vi "Mod_OFDM_Examine_OFDM_Symbol.vi"(0 "Configuration in":variant=variant("Data Source Pool "=variant(cluster{"mode (PN)":enum16{"PN", "pattern", "user"}, "PN sequence order (9)":i32, "base bit pattern (00001111)":enum16{"0", "1", "01", "0011", "00001111"}, "User base bit pattern":i8[]}[] [{"mode (PN)"=enum."PN", "PN sequence order (9)"=9, "base bit pattern (00001111)"=enum."00001111", "User base bit pattern"=[]}, {"mode (PN)"=enum."PN", "PN sequence order (9)"=9, "base bit pattern (00001111)"=enum."00001111", "User base bit pattern"=[]}, {"mode (PN)"=enum."PN", "PN sequence order (9)"=9, "base bit pattern (00001111)"=enum."00001111", "User base bit pattern"=[]}, {"mode (PN)"=enum."PN", "PN sequence order (9)"=9, "base bit pattern (00001111)"=enum."00001111", "User base bit pattern"=[]}, {"mode (PN)"=enum."PN", "PN sequence order (9)"=9, "base bit pattern (00001111)"=enum."00001111", "User base bit pattern"=[]}, {"mode (PN)"=enum."PN", "PN sequence order (9)"=9, "base bit pattern (00001111)"=enum."00001111", "User base bit pattern"=[]}]), "Modulator Source Pool "=variant(cluster{"M-QAM":enum16{"4", "16", "64", "256", "1024"}, "M-PSK":enum16{"2", "4", "8", "16", "32", "64", "128", "256"}, "Type of Modulation":enum16{"PSK", "QAM"}, "PSK":cluster{"differential PSK":enum16{"disable", "enable"}, "PSK type":u16}}[] [{"M-QAM"=enum."4", "M-PSK"=enum."4", "Type of Modulation"=enum."PSK", "PSK"={"differential PSK"=enum."disable", "PSK type"=0}}, {"M-QAM"=enum."4", "M-PSK"=enum."4", "Type of Modulation"=enum."PSK", "PSK"={"differential PSK"=enum."disable", "PSK type"=0}}, {"M-QAM"=enum."4", "M-PSK"=enum."4", "Type of Modulation"=enum."PSK", "PSK"={"differential PSK"=enum."disable", "PSK type"=0}}, {"M-QAM"=enum."4", "M-PSK"=enum."4", "Type of Modulation"=enum."PSK", "PSK"={"differential PSK"=enum."disable", "PSK type"=0}}, {"M-QAM"=enum."4", "M-PSK"=enum."4", "Type of Modulation"=enum."PSK", "PSK"={"differential PSK"=enum."disable", "PSK type"=0}}, {"M-QAM"=enum."4", "M-PSK"=enum."2", "Type of Modulation"=enum."PSK", "PSK"={"differential PSK"=enum."disable", "PSK type"=0}}]), "OFDM SYMBOL POOL"=variant(string[] []), "Sub Carrier Selection"=variant(cluster{"Sub Carrier":bool, "Data Source":u16, "Modulator":u16}[] [{"Sub Carrier"=TRUE, "Data Source"=0, "Modulator"=0}, {"Sub Carrier"=TRUE, "Data Source"=0, "Modulator"=0}, {"Sub Carrier"=TRUE, "Data Source"=0, "Modulator"=0}, {"Sub Carrier"=TRUE, "Data Source"=0, "Modulator"=0}, {"Sub Carrier"=TRUE, "Data Source"=0, "Modulator"=0}, {"Sub Carrier"=TRUE, "Data Source"=0, "Modulator"=0}, {"Sub Carrier"=TRUE, "Data Source"=0, "Modulator"=0}, {"Sub Carrier"=TRUE, "Data Source"=0, "Modulator"=0}, {"Sub Carrier"=TRUE, "Data Source"=0, "Modulator"=0}, {"Sub Carrier"=TRUE, "Data Source"=0, "Modulator"=0}, {"Sub Carrier"=TRUE, "Data Source"=0, "Modulator"=0}, {"Sub Carrier"=TRUE, "Data Source"=0, "Modulator"=0}, {"Sub Carrier"=TRUE, "Data Source"=0, "Modulator"=0}, {"Sub Carrier"=TRUE, "Data Source"=0, "Modulator"=0}, {"Sub Carrier"=TRUE, "Data Source"=0, "Modulator"=0}, {"Sub Carrier"=TRUE, "Data Source"=0, "Modulator"=0}, {"Sub Carrier"=TRUE, "Data Source"=0, "Modulator"=0}, {"Sub Carrier"=TRUE, "Data Source"=0, "Modulator"=0}, {"Sub Carrier"=TRUE, "Data Source"=0, "Modulator"=0}, {"Sub Carrier"=TRUE, "Data Source"=0, "Modulator"=0}, {"Sub Carrier"=TRUE, "Data Source"=0, "Modulator"=0}, {"Sub Carrier"=TRUE, "Data Source"=0, "Modulator"=0}, {"Sub Carrier"=TRUE, "Data Source"=0, "Modulator"=0}, {"Sub Carrier"=TRUE, "Data Source"=0, "Modulator"=0}, {"Sub Carrier"=TRUE, "Data Source"=0, "Modulator"=0}, {"Sub Carrier"=TRUE, "Data Source"=0, "Modulator"=0}, {"Sub Carrier"=TRUE, "Data Source"=0, "Modulator"=0}, {"Sub Carrier"=TRUE, "Data Source"=0, "Modulator"=0}, {"Sub Carrier"=TRUE, "Data Source"=0, "Modulator"=0}, {"Sub Carrier"=TRUE, "Data Source"=0, "Modulator"=0}, {"Sub Carrier"=TRUE, "Data Source"=0, "Modulator"=0}, {"Sub Carrier"=TRUE, "Data Source"=0, "Modulator"=0}, {"Sub Carrier"=TRUE, "Data Source"=0, "Modulator"=0}, {"Sub Carrier"=TRUE, "Data Source"=0, "Modulator"=0}, {"Sub Carrier"=TRUE, "Data Source"=0, "Modulator"=0}, {"Sub Carrier"=TRUE, "Data Source"=0, "Modulator"=0}, {"Sub Carrier"=TRUE, "Data Source"=0, "Modulator"=0}, {"Sub Carrier"=TRUE, "Data Source"=0, "Modulator"=0}, {"Sub Carrier"=TRUE, "Data Source"=0, "Modulator"=0}, {"Sub Carrier"=TRUE, "Data Source"=0, "Modulator"=0}, {"Sub Carrier"=TRUE, "Data Source"=0, "Modulator"=0}, {"Sub Carrier"=TRUE, "Data Source"=0, "Modulator"=0}, {"Sub Carrier"=TRUE, "Data Source"=0, "Modulator"=0}, {"Sub Carrier"=TRUE, "Data Source"=0, "Modulator"=0}, {"Sub Carrier"=TRUE, "Data Source"=0, "Modulator"=0}, {"Sub Carrier"=TRUE, "Data Source"=0, "Modulator"=0}, {"Sub Carrier"=TRUE, "Data Source"=0, "Modulator"=0}, {"Sub Carrier"=TRUE, "Data Source"=0, "Modulator"=0}, {"Sub Carrier"=TRUE, "Data Source"=0, "Modulator"=0}, {"Sub Carrier"=TRUE, "Data Source"=0, "Modulator"=0}, {"Sub Carrier"=TRUE, "Data Source"=0, "Modulator"=0}, {"Sub Carrier"=TRUE, "Data Source"=0, "Modulator"=0}, {"Sub Carrier"=TRUE, "Data Source"=0, "Modulator"=0}, {"Sub Carrier"=TRUE, "Data Source"=0, "Modulator"=0}, {"Sub Carrier"=TRUE, "Data Source"=0, "Modulator"=0}, {"Sub Carrier"=TRUE, "Data Source"=0, "Modulator"=0}, {"Sub Carrier"=TRUE, "Data Source"=0, "Modulator"=0}, {"Sub Carrier"=TRUE, "Data Source"=0, "Modulator"=0}, {"Sub Carrier"=TRUE, "Data Source"=0, "Modulator"=0}, {"Sub Carrier"=TRUE, "Data Source"=0, "Modulator"=0}, {"Sub Carrier"=TRUE, "Data Source"=0, "Modulator"=0}, {"Sub Carrier"=TRUE, "Data Source"=0, "Modulator"=0}, {"Sub Carrier"=TRUE, "Data Source"=0, "Modulator"=0}, {"Sub Carrier"=TRUE, "Data Source"=0, "Modulator"=0}, {"Sub Carrier"=TRUE, "Data Source"=0, "Modulator"=0}, {"Sub Carrier"=TRUE, "Data Source"=0, "Modulator"=0}, {"Sub Carrier"=TRUE, "Data Source"=0, "Modulator"=0}, {"Sub Carrier"=TRUE, "Data Source"=0, "Modulator"=0}, {"Sub Carrier"=TRUE, "Data Source"=0, "Modulator"=0}, {"Sub Carrier"=TRUE, "Data Source"=0, "Modulator"=0}, {"Sub Carrier"=TRUE, "Data Source"=0, "Modulator"=0}, {"Sub Carrier"=TRUE, "Data Source"=0, "Modulator"=0}, {"Sub Carrier"=TRUE, "Data Source"=0, "Modulator"=0}, {"Sub Carrier"=TRUE, "Data Source"=0, "Modulator"=0}, {"Sub Carrier"=TRUE, "Data Source"=0, "Modulator"=0}, {"Sub Carrier"=TRUE, "Data Source"=0, "Modulator"=0}, {"Sub Carrier"=TRUE, "Data Source"=0, "Modulator"=0}, {"Sub Carrier"=TRUE, "Data Source"=0, "Modulator"=0}, {"Sub Carrier"=TRUE, "Data Source"=0, "Modulator"=0}, {"Sub Carrier"=TRUE, "Data Source"=0, "Modulator"=0}, {"Sub Carrier"=TRUE, "Data Source"=0, "Modulator"=0}, {"Sub Carrier"=TRUE, "Data Source"=0, "Modulator"=0}, {"Sub Carrier"=TRUE, "Data Source"=0, "Modulator"=0}, {"Sub Carrier"=TRUE, "Data Source"=0, "Modulator"=0}, {"Sub Carrier"=TRUE, "Data Source"=0, "Modulator"=0}, {"Sub Carrier"=TRUE, "Data Source"=0, "Modulator"=0}, {"Sub Carrier"=TRUE, "Data Source"=0, "Modulator"=0}, {"Sub Carrier"=TRUE, "Data Source"=0, "Modulator"=0}, {"Sub Carrier"=TRUE, "Data Source"=0, "Modulator"=0}, {"Sub Carrier"=TRUE, "Data Source"=0, "Modulator"=0}, {"Sub Carrier"=TRUE, "Data Source"=0, "Modulator"=0}, {"Sub Carrier"=TRUE, "Data Source"=0, "Modulator"=0}, {"Sub Carrier"=TRUE, "Data Source"=0, "Modulator"=0}, {"Sub Carrier"=TRUE, "Data Source"=0, "Modulator"=0}, {"Sub Carrier"=TRUE, "Data Source"=0, "Modulator"=0}, {"Sub Carrier"=TRUE, "Data Source"=0, "Modulator"=0}, {"Sub Carrier"=TRUE, "Data Source"=0, "Modulator"=0}, {"Sub Carrier"=TRUE, "Data Source"=0, "Modulator"=0}, {"Sub Carrier"=TRUE, "Data Source"=0, "Modulator"=0}, {"Sub Carrier"=TRUE, "Data Source"=0, "Modulator"=0}, {"Sub Carrier"=TRUE, "Data Source"=0, "Modulator"=0}, {"Sub Carrier"=TRUE, "Data Source"=0, "Modulator"=0}, {"Sub Carrier"=TRUE, "Data Source"=0, "Modulator"=0}, {"Sub Carrier"=TRUE, "Data Source"=0, "Modulator"=0}, {"Sub Carrier"=TRUE, "Data Source"=0, "Modulator"=0}, {"Sub Carrier"=TRUE, "Data Source"=0, "Modulator"=0}, {"Sub Carrier"=TRUE, "Data Source"=0, "Modulator"=0}, {"Sub Carrier"=TRUE, "Data Source"=0, "Modulator"=0}, {"Sub Carrier"=TRUE, "Data Source"=0, "Modulator"=0}, {"Sub Carrier"=TRUE, "Data Source"=0, "Modulator"=0}, {"Sub Carrier"=TRUE, "Data Source"=0, "Modulator"=0}, {"Sub Carrier"=TRUE, "Data Source"=0, "Modulator"=0}, {"Sub Carrier"=TRUE, "Data Source"=0, "Modulator"=0}, {"Sub Carrier"=TRUE, "Data Source"=0, "Modulator"=0}, {"Sub Carrier"=TRUE, "Data Source"=0, "Modulator"=0}, {"Sub Carrier"=TRUE, "Data Source"=0, "Modulator"=0}, {"Sub Carrier"=TRUE, "Data Source"=0, "Modulator"=0}, {"Sub Carrier"=TRUE, "Data Source"=0, "Modulator"=0}, {"Sub Carrier"=TRUE, "Data Source"=0, "Modulator"=0}, {"Sub Carrier"=TRUE, "Data Source"=0, "Modulator"=0}, {"Sub Carrier"=TRUE, "Data Source"=0, "Modulator"=0}, {"Sub Carrier"=TRUE, "Data Source"=0, "Modulator"=0}, {"Sub Carrier"=TRUE, "Data Source"=0, "Modulator"=0}, {"Sub Carrier"=TRUE, "Data Source"=0, "Modulator"=0}, {"Sub Carrier"=TRUE, "Data Source"=0, "Modulator"=0}, {"Sub Carrier"=TRUE, "Data Source"=0, "Modulator"=0}, {"Sub Carrier"=TRUE, "Data Source"=0, "Modulator"=0}, {"Sub Carrier"=TRUE, "Data Source"=0, "Modulator"=0}]), "Symbol Table"=variant(string[][] [])), 11 "error in":errorcluster) -> (3 "Data Source Names":string[](array[string]), 4 "Configuration out":variant, 6 "OFDM Parameters":T1, 8 "DATA Source Pool":T2 {"Register Initial State" format="%08x"}, 10 "Modulator Pool":T3, 14 "Mod Names":string[](array[string]), 15 "error out":errorcluster)   [LabVIEW 2010]
uses:
  Controls(Type_DEf)/Pool of Modulator Control.ctl
  Controls(Type_DEf)/Pool of Data Source Control.ctl
  Polymorphic_Sub_VI's/Mod_OFDM_Get_Data_Sources.vi
  Polymorphic_Sub_VI's/Mod_OFDM_Get_Modulator_Sources.vi
  Polymorphic_Sub_VI's/Mod_OFDM_Get_Ofdm_Parameters.vi
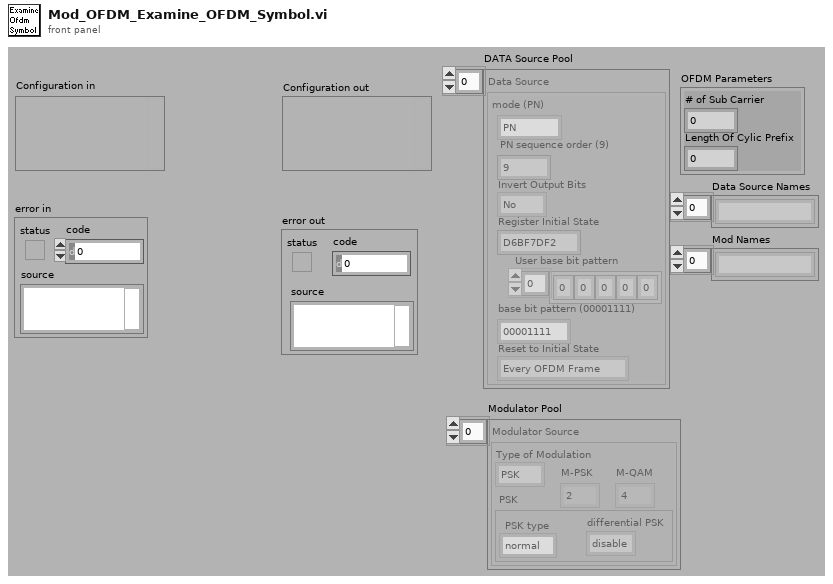
[diagram p1: front panel]
types:
  T1 = cluster{"# of Sub Carrier":i32, "Length Of Cylic Prefix":i32}
  T2 = typedef "Pool of Data Source Control.ctl" = cluster{"mode (PN)":enum16{"PN", "pattern", "user"}, "PN sequence order (9)":i32, "Invert Output Bits":enum16{"No", "Yes"}, "Register Initial State ":u32, "User base bit pattern":i8[], "base bit pattern (00001111)":enum16{"0", "1", "01", "0011", "00001111"}, "Reset to Initial State":enum16{"Every OFDM Frame", "Every OFDM Symbol", "Every Sub Carrier"}}[]
  T3 = typedef "Pool of Modulator Control.ctl" = cluster{"M-QAM":enum16{"4", "16", "64", "256"}, "M-PSK":enum16{"2", "4", "8", "16", "32", "64", "128", "256"}, "Type of Modulation":enum16{"PSK", "QAM"}, " PSK":cluster{"differential PSK":enum16{"disable", "enable"}, "PSK type":enum16{"normal", "shifted", "offset"}}}[]
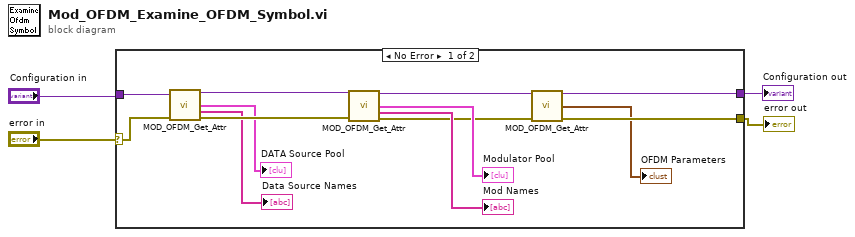
[diagram p0: block diagram]
diagram:
  n1 = case shown="No Error" "error in" {
    selector: "error in" -> [w11 w18]
    tunnel: "Configuration in" -> [w10 _]
    tunnel: [w7 _] -> w3
    tunnel: [w6 w18] -> w1
    frame No Error {
      n2 = call-poly "MOD_OFDM_Get_Attr.vi"("Configuration in"=w10, "error in"=w11) -> ("Configuration out"=w17:variant, "Pool of Data Sources"=→"DATA Source Pool":T2, "Data Source Names"=→"Data Source Names":string[], "error out"=w16:errorcluster)  [unwired: 7 in, 3 out]
      n3 = call-poly "MOD_OFDM_Get_Attr.vi"("Configuration in"=w17, "error in"=w16) -> ("Configuration out"=w8:variant, "Pool of Modulators"=→"Modulator Pool":T3, "Modulator Source Names"=→"Mod Names":string[], "error out"=w9:errorcluster)  [unwired: 8 in, 2 out]
      n4 = call-poly "MOD_OFDM_Get_Attr.vi"("Configuration in"=w8, "error in"=w9) -> ("Configuration out"=w7:variant, "OFDM Parameters"=→"OFDM Parameters":T1, "error out"=w6:errorcluster)  [unwired: 10 in, 1 out]
    }
    frame Error {
    }
  }
  "error out" <- w1
  "Configuration out" <- w3
